vi "IMS Stepper Move.vi"(4 "Mode":bool, 5 "error in (no error)":errorcluster, 6 "Distance":dbl=1.0 min=-193273528.32 max=193273528.0 step=0.09 format="%.2f", 7 "Motor Number":u32=1 min=1 max=255 step=1, 8 "Instrument Address":refnum<visa-resource-name>) -> (0 "error out":errorcluster, 3 "Instrument Address Out":refnum<visa-resource-name>)   [LabVIEW 2019]
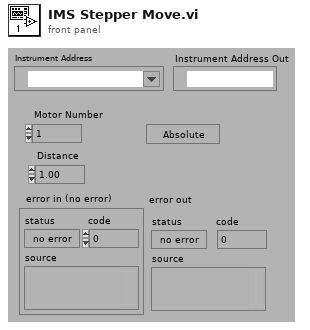
[diagram p1: front panel]
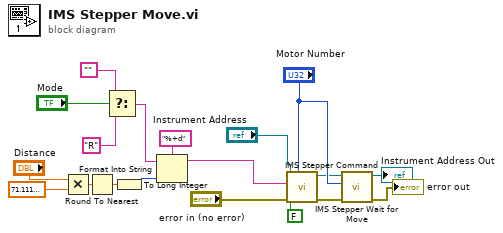
[diagram p0: block diagram]
diagram:
  n1 = Multiply(x="Distance", y=71.11111111) -> (x*y=w17:dbl)
  n2 = Round To Nearest(number=w17) -> (nearest integer value=w15:dbl)
  n3 = Select(t="", s="Mode", f="R") -> (s? t:f=w7:string)
  n4 = To Long Integer(number=w15) -> (32bit integer=w16:i32)
  n5 = Format Into String(format string="%+d", initial string=w7, w16) -> (resulting string=w6:string)  [unwired: 1 in, 1 out]
  n6 = call "IMS Stepper Command.vi"("Motor Number"="Motor Number", "error in (no error)"="error in (no error)", "Mode"=FALSE, "Command"=w6, "Instrument Address"="Instrument Address") -> ("error out"=w12:errorcluster, "Instrument Address Out"=w2:refnum<visa-resource-name>)  [unwired: 1 in, 2 out]
  n7 = call "IMS Stepper Wait for Move.vi"("error in (no error)"=w12, "Motor Number"="Motor Number", "Instrument Address"=w2) -> ("error out"=→"error out":errorcluster, "Instrument Address Out"=→"Instrument Address Out":refnum<visa-resource-name>)  [unwired: 4 in]
